vi "DualMotorControl_v2.vi"() -> ()   [LabVIEW 2019]
uses:
  <vilib>/myRIO/Common/Instrument Driver Framework/myRIO v1.0/Encoder/typedefs/Encoder Signal Mode.ctl
  <vilib>/myRIO/Instrument Drivers/Onboard IO/Encoder/typedefs/Encoder Reference.ctl
  <vilib>/myRIO/Common/Instrument Driver Framework/Utilities/typedefs/myRIO Generic Hardware Reference.ctl
  <vilib>/myRIO/Common/Instrument Driver Framework/Utilities/typedefs/Hardware Version Enum.ctl
  <vilib>/myRIO/Common/Instrument Driver Framework/Utilities/typedefs/myRIO v1.0 Reference.ctl
  <vilib>/myRIO/Common/Instrument Driver Framework/Utilities/typedefs/Generic FPGA Reference.ctl
  <vilib>/myRIO/Common/Instrument Driver Framework/myRIO v1.0/Encoder/typedefs/Encoder Channels Enum.ctl
  <vilib>/myRIO/Common/Instrument Driver Framework/myRIO v1.0/Encoder/typedefs/Encoder Configuration v1.0.ctl
  <vilib>/userDefined/High Color/nirio_resource_hc.ctl
  <vilib>/Platform/TimedLoop/XDataNode/timing_clust.ctl
  <vilib>/Platform/TimedLoop/XDataNode/nitl_modes.ctl
  <vilib>/Platform/TimedLoop/XDataNode/wakeup.ctl
  <vilib>/myRIO/Instrument Drivers/Onboard IO/PWM/typedefs/PWM Reference.ctl
  <vilib>/myRIO/Common/Instrument Driver Framework/myRIO v1.0/PWM/typedefs/PWM Channels Enum.ctl
  <vilib>/myRIO/Instrument Drivers/Onboard IO/PWM/typedefs/PWM Configuration.ctl
  <vilib>/myRIO/Instrument Drivers/Onboard IO/DIO/typedefs/DIO Reference.ctl
  <vilib>/myRIO/Common/Instrument Driver Framework/myRIO v1.0/DIO/typedefs/DIO Channels List.ctl
  <vilib>/myRIO/Common/Instrument Driver Framework/myRIO v1.0/DIO/typedefs/DIO Channels Enum.ctl
  <vilib>/myRIO/Common/Instrument Driver Framework/Utilities/vis/Is FPGA Ref Available.vi
  <vilib>/myRIO/Common/Instrument Driver Framework/myRIO v1.0/Encoder/vis/myRIO v1.1 Open Encoder.vi
  <vilib>/myRIO/Instrument Drivers/Onboard IO/Encoder/vis/Read.vi
  <vilib>/myRIO/Common/Instrument Driver Framework/myRIO v1.0/PWM/vis/myRIO v1.1 Open PWM.vi
  <vilib>/myRIO/Instrument Drivers/Onboard IO/PWM/vis/Set Duty Cycle and Frequency.vi
  <vilib>/myRIO/Common/Instrument Driver Framework/myRIO v1.0/DIO/vis/myRIO v1.1 Open DIO.vi
  <vilib>/myRIO/Instrument Drivers/Onboard IO/DIO/vis/Write.vi
  <vilib>/myRIO/Common/Instrument Driver Framework/Utilities/vis/Validate Channels.vi
  <vilib>/myRIO/Common/Instrument Driver Framework/myRIO v1.0/Encoder/vis/myRIO v1.0 Reserve Encoder.vi
  <vilib>/myRIO/Common/Instrument Driver Framework/myRIO v1.0/PWM/vis/myRIO v1.0 Reserve PWM.vi
  <vilib>/myRIO/Common/Instrument Driver Framework/myRIO v1.0/DIO/vis/myRIO v1.0 Reserve DIO.vi
  <vilib>/myRIO/Common/Instrument Driver Framework/myRIO v1.0/Encoder/vis/myRIO v1.0 Build MUX Configuration Encoder.vi
  <vilib>/myRIO/Common/Instrument Driver Framework/myRIO v1.0/Resource Manager/vis/myRIO v1.0 Reserve Channel List.vi
  <vilib>/myRIO/Common/Instrument Driver Framework/myRIO v1.0/PWM/vis/myRIO v1.0 Build MUX Configuration PWM.vi
  <vilib>/myRIO/Common/Instrument Driver Framework/myRIO v1.0/DIO/vis/myRIO v1.0 Build MUX Configuration DIO.vi
  <vilib>/myRIO/Common/Instrument Driver Framework/myRIO v1.0/Resource Manager/vis/myRIO v1.0 Create Configuration List.vi
  <vilib>/myRIO/Common/Instrument Driver Framework/myRIO v1.0/Resource Manager/vis/myRIO v1.0 Reserve Channel.vi
  <vilib>/myRIO/Common/Instrument Driver Framework/myRIO v1.0/Resource Manager/vis/myRIO v1.0 Unreserve Channel.vi
  <vilib>/myRIO/Common/Instrument Driver Framework/myRIO v1.0/Resource Manager/vis/myRIO v1.0 Build Mutex Name.vi
  <vilib>/Utility/VariantDataType/GetNumericInfo.vi
  <vilib>/Utility/error.llb/Error Cluster From Error Code.vi
  <vilib>/myRIO/Common/Instrument Driver Framework/myRIO v1.0/myRIO v1.1 Open.vi
  <vilib>/myRIO/Common/Instrument Driver Framework/Utilities/vis/IO Manager.vi
  <vilib>/myRIO/Common/Instrument Driver Framework/Utilities/vis/Configuration Manager.vi
  <vilib>/myRIO/Common/Instrument Driver Framework/myRIO v1.0/Resource Manager/vis/myRIO v1.0 Configure IO.vi
  <vilib>/myRIO/Common/Instrument Driver Framework/myRIO v1.0/myRIO v1.0 Close.vi
  <vilib>/myRIO/Common/Instrument Driver Framework/myRIO v1.0/Encoder/vis/myRIO v1.0 Configure Encoder.vi
  <vilib>/myRIO/Common/Instrument Driver Framework/myRIO v1.0/Encoder/vis/myRIO v1.0 Read Encoder.vi
  <vilib>/Instr/_visa.llb/VISA Configure Serial Port (Instr).vi
  <vilib>/myRIO/Common/Instrument Driver Framework/myRIO v1.0/PWM/vis/myRIO v1.0 Write PWM.vi
  <vilib>/myRIO/Common/Instrument Driver Framework/myRIO v1.0/DIO/vis/myRIO v1.0 Write DIO.vi
  <vilib>/Utility/file.llb/Write Delimited Spreadsheet (DBL).vi
  <vilib>/myRIO/Express VI/Onboard IO/Encoder/Encoder Express VI.xnode
  <vilib>/myRIO/Instrument Drivers/Onboard IO/Encoder/vis/myRIO Encoder Open.xnode
  <vilib>/myRIO/Common/Instrument Driver Framework/myRIO v1.0/Encoder/typedefs/Encoder Count Direction Enum.ctl
  <vilib>/Platform/TimedLoop/XDataNode/XDataNode.xnode
  <vilib>/myRIO/Express VI/Onboard IO/PWM/PWM Express VI.xnode
  <vilib>/myRIO/Instrument Drivers/Onboard IO/PWM/vis/myRIO PWM Open.xnode
  <vilib>/myRIO/Express VI/Onboard IO/DO/DO Express VI.xnode
  <vilib>/myRIO/Instrument Drivers/Onboard IO/DIO/vis/myRIO DIO Open.xnode
  <vilib>/myRIO/Instrument Drivers/Onboard IO/Encoder/Encoder.lvlib
  <vilib>/Platform/TimedLoop/XDataNode/XDNodeRunTimeDep.lvlib
  <vilib>/myRIO/Instrument Drivers/Onboard IO/PWM/PWM.lvlib
  <vilib>/myRIO/Instrument Drivers/Onboard IO/DIO/DIO.lvlib
panel:
  out "element":string
  in  "Encoder_Count":dbl=54991.0
  out "number":i32
  in  "text":string[](array[string])
  in  "start FIFO":bool=TRUE
  out "Write FIFO error":errorcluster
  out "# elements write":u32=219
  out "timed out?":bool
  out "rt fifo":refnum<k33>
  in  "Buffer factor":dbl=1.5
  out "# elements read":u32
  out "date/time string":string="1970011"
  out "Create FIFO error":errorcluster
  in  "Experiment Mode":string="20250310_servo_sinewave"
  in  "Times":string="0"
  in  "File Path Control":path=path "C:/Rhex_ABAD"
  out "error out":errorcluster
  in  "baud rate (9600)":u32=500000
  in  "VISA resource name":refnum<visa-resource-name>="ASRL2::INSTR"
  in  "stop":bool
  in  "const posotion":dbl=180.0
  out "write to visa":string
  out "read from visa":string
  out "sine position":dbl
  out "time":dbl
  out "iteration":i32
  in  "const(f)/sine(t)":bool
  in  "sinewave period":dbl=10.0
  in  "Gain":T1={"P Gain"=0.5, "I Gain"=0.0, "D Gain"=0.005}
  in  "Frequency":dbl=1000.0
  out "Duty cycle  2":dbl
  in  "Loop Period":i64=5
  # "Servo motor"
  # "Control botton"
  # "Plot"
  # "visa setting"
  # "servo setting"
  # "Timed loop status"
  # "DC motor"
  # "R-SLIP Parameters"
  # "v = 1; a = 15"
  # "v = 1.25; a = 15"
  # "v = 1.5; a = 15"
  # "0.184067181524967\n0.263820978418769\n256152.551336786\n-30272.30000274\n-9876.03760433421\n-1096.38594197941\n885.91817900106\n-44.6781799901984"
  # "0.215241998794118\n0.254514142390288\n4771.41078363533\n62185.8763006578\n-22508.5336527453\n390.805502041188\n686.695311017595\n-40.4128145310291"
  # "0.163616269216122\n0.27489641502463\n771965.39318528\n-201617.027694185\n8828.08396944145\n-2683.04589908678\n1085.57303422127\n-48.5860395324432"
  # "v = 1.75; a = 15"
  # "v = 2; a = 15"
  # "v = 2.25; a = 15"
  # "0.148651048423414\n0.288542414074344\n1776973.44893281\n-511591.467559457\n38775.9830765103\n-4576.94506688942\n1289.39828252671\n-52.3115561007577"
  # "0.136976185169818\n0.304016701267508\n3461279.85083822\n-993110.73746345\n80544.6579529191\n-6699.48295844177\n1494.82265451498\n-55.8934424469099"
  # "0.134381902205816\n0.369022171779704\n3272804.8365432\n-899365.569589567\n71225.2463409934\n-7039.10791102172\n1512.66147498591\n-59.3408899720725"
  # "FIFO status"
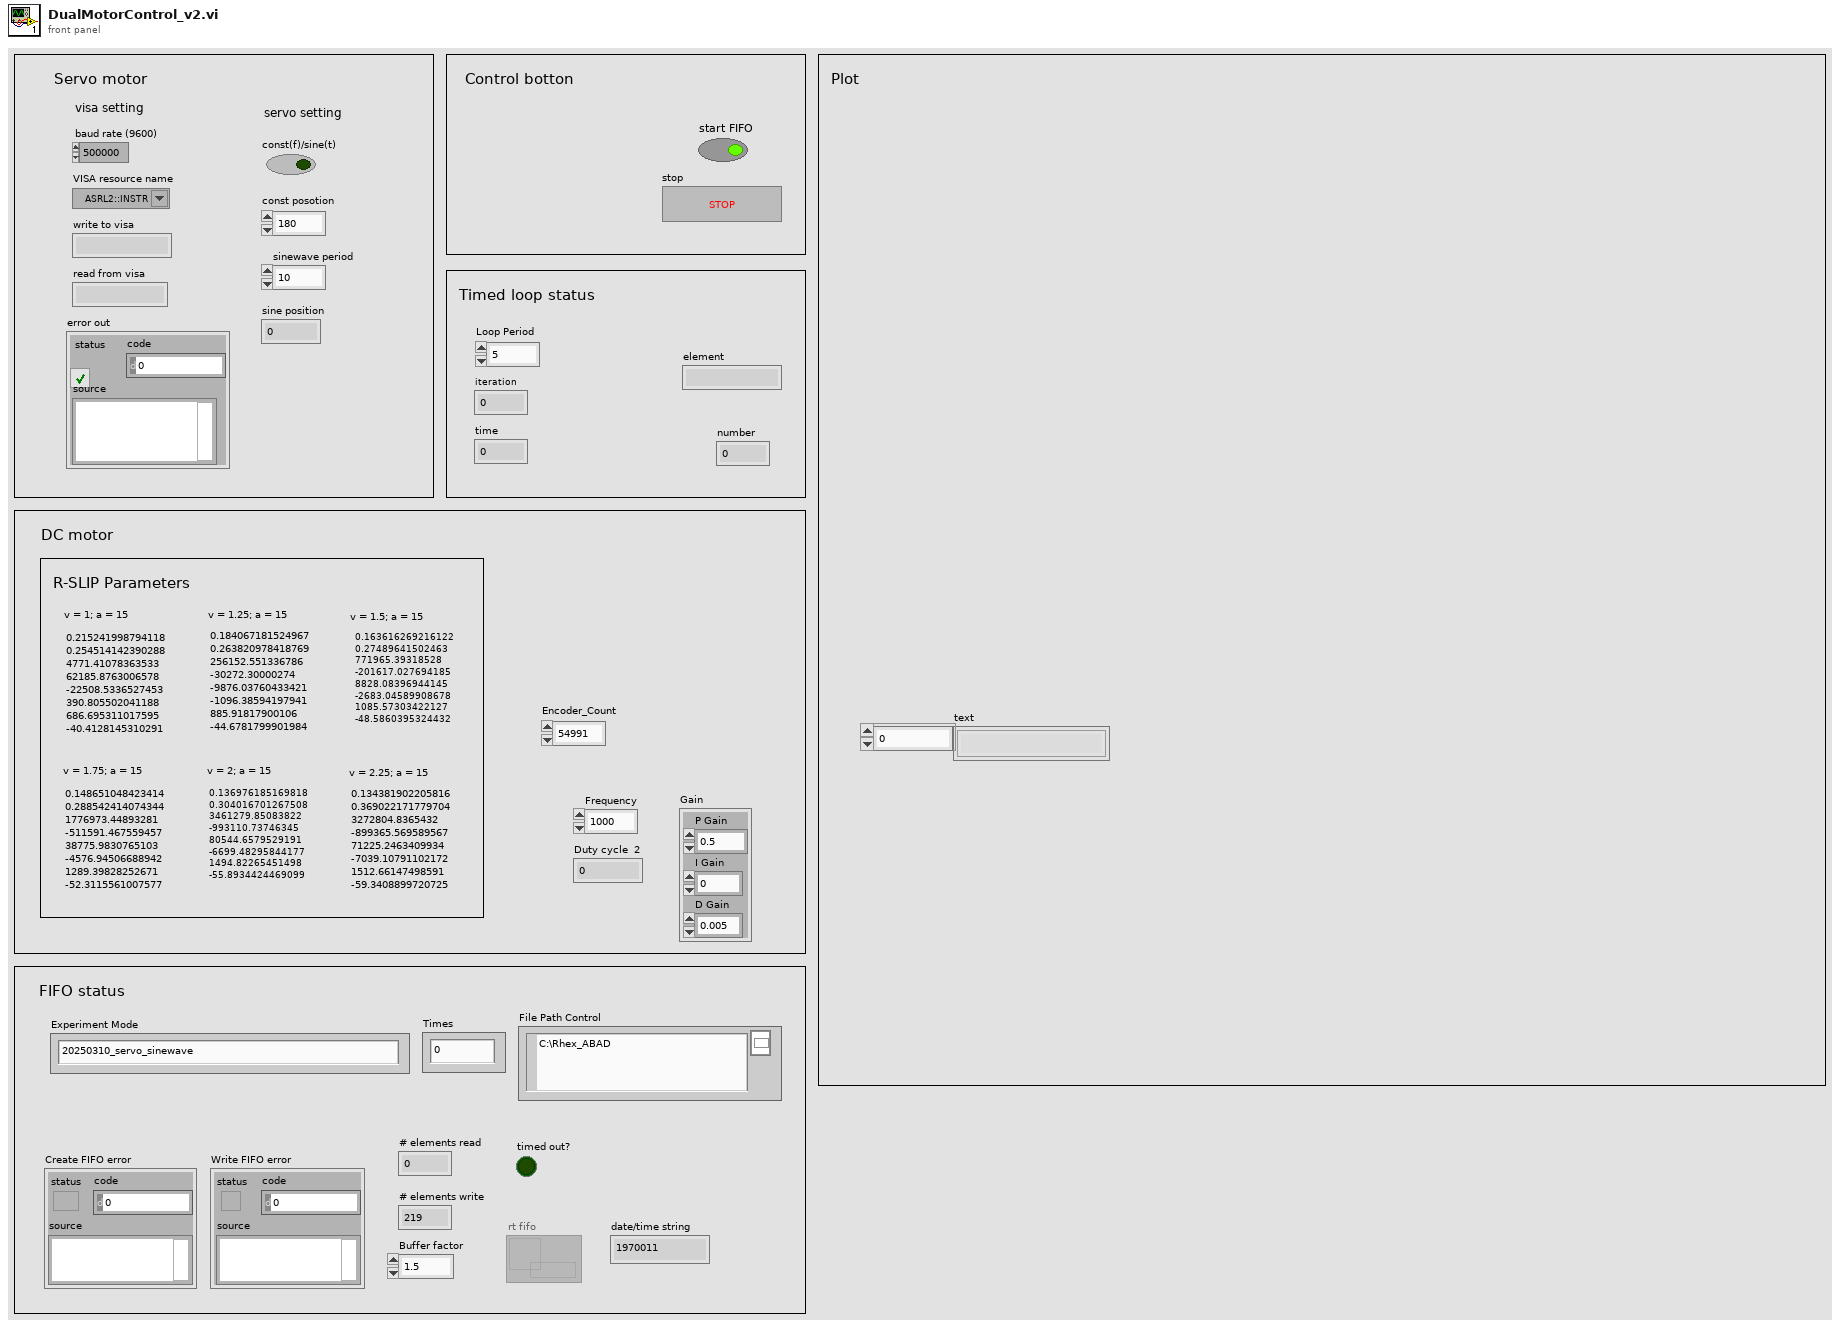
[diagram p1: front panel]
types:
  T1 = cluster{"P Gain":dbl, "I Gain":dbl, "D Gain":dbl}
  T2 = typedef "Encoder.lvlib/Encoder Reference.ctl" = cluster{"myRIO Reference":T3, "Encoder Channels Enum":T7}
  T3 = typedef "myRIO Generic Hardware Reference.ctl" = cluster{"myRIO Model":T4, "myRIO Hardware Reference":T5}
  T4 = typedef "Hardware Version Enum.ctl" = enum16{"Unknown", "myRIO-1900", "myRIO-1950", "roboRIO", "NI ELVIS RIO CM", "ELVIS III"}
  T5 = typedef "myRIO v1.0 Reference.ctl" = cluster{"Generic FPGA Reference":T6, "Allow multiple opens":bool}
  T6 = typedef "Generic FPGA Reference.ctl" = refnum<k20>
  T7 = typedef "Encoder Channels Enum.ctl" = enum16{"Not Connected", "C/ENC0", "C/ENC1", "A/ENC", "A/ENC0", "A/ENC1", "A/ENC2", "A/ENC3", "A/ENC4", "A/ENC5", "A/ENC6", "A/ENC7", "A/ENC8", "A/ENC9", "B/ENC", "B/ENC0", "B/ENC1", "B/ENC2", "B/ENC3", "B/ENC4", "B/ENC5", "B/ENC6", "B/ENC7", "B/ENC8", "B/ENC9", "DIO/ENC0", "DIO/ENC1", "DIO/ENC2", "DIO/ENC3", "DIO/ENC4"}
  T8 = typedef "Encoder Signal Mode.ctl" = enum16{"Quadrature phase signal", "Step and direction signal"}
  T9 = typedef "nirio_resource_hc.ctl" = tag
  T10 = typedef "DIO.lvlib/DIO Reference.ctl" = cluster{"myRIO Reference":T3, "DIO Channels List":T11}
  T11 = typedef "DIO Channels List.ctl" = T12[]
  T12 = typedef "DIO Channels Enum.ctl" = enum16{"Not Connected", "C/DIO0", "C/DIO1", "C/DIO2", "C/DIO3", "C/DIO4", "C/DIO5", "C/DIO6", "C/DIO7", "A/DIO0", "A/DIO1", "A/DIO2", "A/DIO3", "A/DIO4", "A/DIO5", "A/DIO6", "A/DIO7", "A/DIO8", "A/DIO9", "A/DIO10", "A/DIO11", "A/DIO12", "A/DIO13", "A/DIO14", "A/DIO15", "A/DIO16", "A/DIO17", "A/DIO18", "A/DIO19", "B/DIO0", "B/DIO1", "B/DIO2", "B/DIO3", "B/DIO4", "B/DIO5", "B/DIO6", "B/DIO7", "B/DIO8", "B/DIO9", "B/DIO10", "B/DIO11", "B/DIO12", "B/DIO13", "B/DIO14", "B/DIO15", "B/DIO16", "B/DIO17", "B/DIO18", "B/DIO19", "LED0", "LED1", "LED2", "LED3", "Button0", "DIO/DIO0", "DIO/DIO1", "DIO/DIO2", "DIO/DIO3", "DIO/DIO4", "DIO/DIO5", "DIO/DIO6", "DIO/DIO7", "DIO/DIO8", "DIO/DIO9", "SPI/CS0", "SPI/CS1", "SPI/CS2", "SPI/CS3", "LED RADIO (Green)", "LED RADIO (Red)", "LED COMM (Green)", "LED COMM (Red)", "LED MODE (Green)", "LED MODE (Red)"}
  T13 = typedef "PWM.lvlib/PWM Reference.ctl" = cluster{"myRIO Reference":T3, "PWM Channels Enum":T14, "PWM Configuration":T15}
  T14 = typedef "PWM Channels Enum.ctl" = enum16{"Not Connected", "C/PWM0", "C/PWM1", "A/PWM0", "A/PWM1", "A/PWM2", "A/PWM3", "A/PWM4", "A/PWM5", "A/PWM6", "A/PWM7", "A/PWM8", "A/PWM9", "A/PWM10", "A/PWM11", "A/PWM12", "A/PWM13", "A/PWM14", "A/PWM15", "A/PWM16", "A/PWM17", "A/PWM18", "A/PWM19", "B/PWM0", "B/PWM1", "B/PWM2", "B/PWM3", "B/PWM4", "B/PWM5", "B/PWM6", "B/PWM7", "B/PWM8", "B/PWM9", "B/PWM10", "B/PWM11", "B/PWM12", "B/PWM13", "B/PWM14", "B/PWM15", "B/PWM16", "B/PWM17", "B/PWM18", "B/PWM19", "PWM/PWM0", "PWM/PWM1", "PWM/PWM2", "PWM/PWM3", "PWM/PWM4", "PWM/PWM5", "PWM/PWM6", "PWM/PWM7", "PWM/PWM8", "PWM/PWM9"}
  T15 = typedef "PWM.lvlib/PWM Configuration.ctl" = cluster{"Frequency":dbl, "Duty Cycle":dbl}
  T16 = typedef "XDNodeRunTimeDep.lvlib/timing_clust.ctl" = cluster{"Expected End [f-1]":u64, "Actual End [f-1]":u64, "Finished Late? [f-1]":bool, "Expected End [i-1]":u64, "Actual End [i-1]":u64, "Finished Late? [i-1]":bool, "Expected Start [i]":u64, "Actual Start [i]":u64, "Expected Start [f]":u64, "Actual Start [f]":u64, "Source Name":string, "Structure Name":string, "Period":i64, "Deadline":i64, "Offset":i64, "Start":i64, "Priority":i32, "Timeout":i32, "Mode":T17, "Wakeup Reason":T18, "Error":errorcluster, "Source Type":string, "Secondary Source Type":string, "Global End Time":u64, "Global Start Time":u64, "Frame Duration":u64, "Iteration Duration":u64, "Assigned CPU":i32, "I/O Scan Engine Mode":u32}
  T17 = typedef "XDNodeRunTimeDep.lvlib/nitl_modes.ctl" = enum32{"No Change", "Process missed periods, maintain original phase", "Discard missed periods, maintain original phase", "Process missed periods, ignore original phase", "Discard missed periods, ignore original phase"}
  T18 = typedef "XDNodeRunTimeDep.lvlib/wakeup.ctl" = enum32{"Normal", "Aborted", "Asynchronous wakeup", "Timing source error", "Timed loop error", "Timeout"}
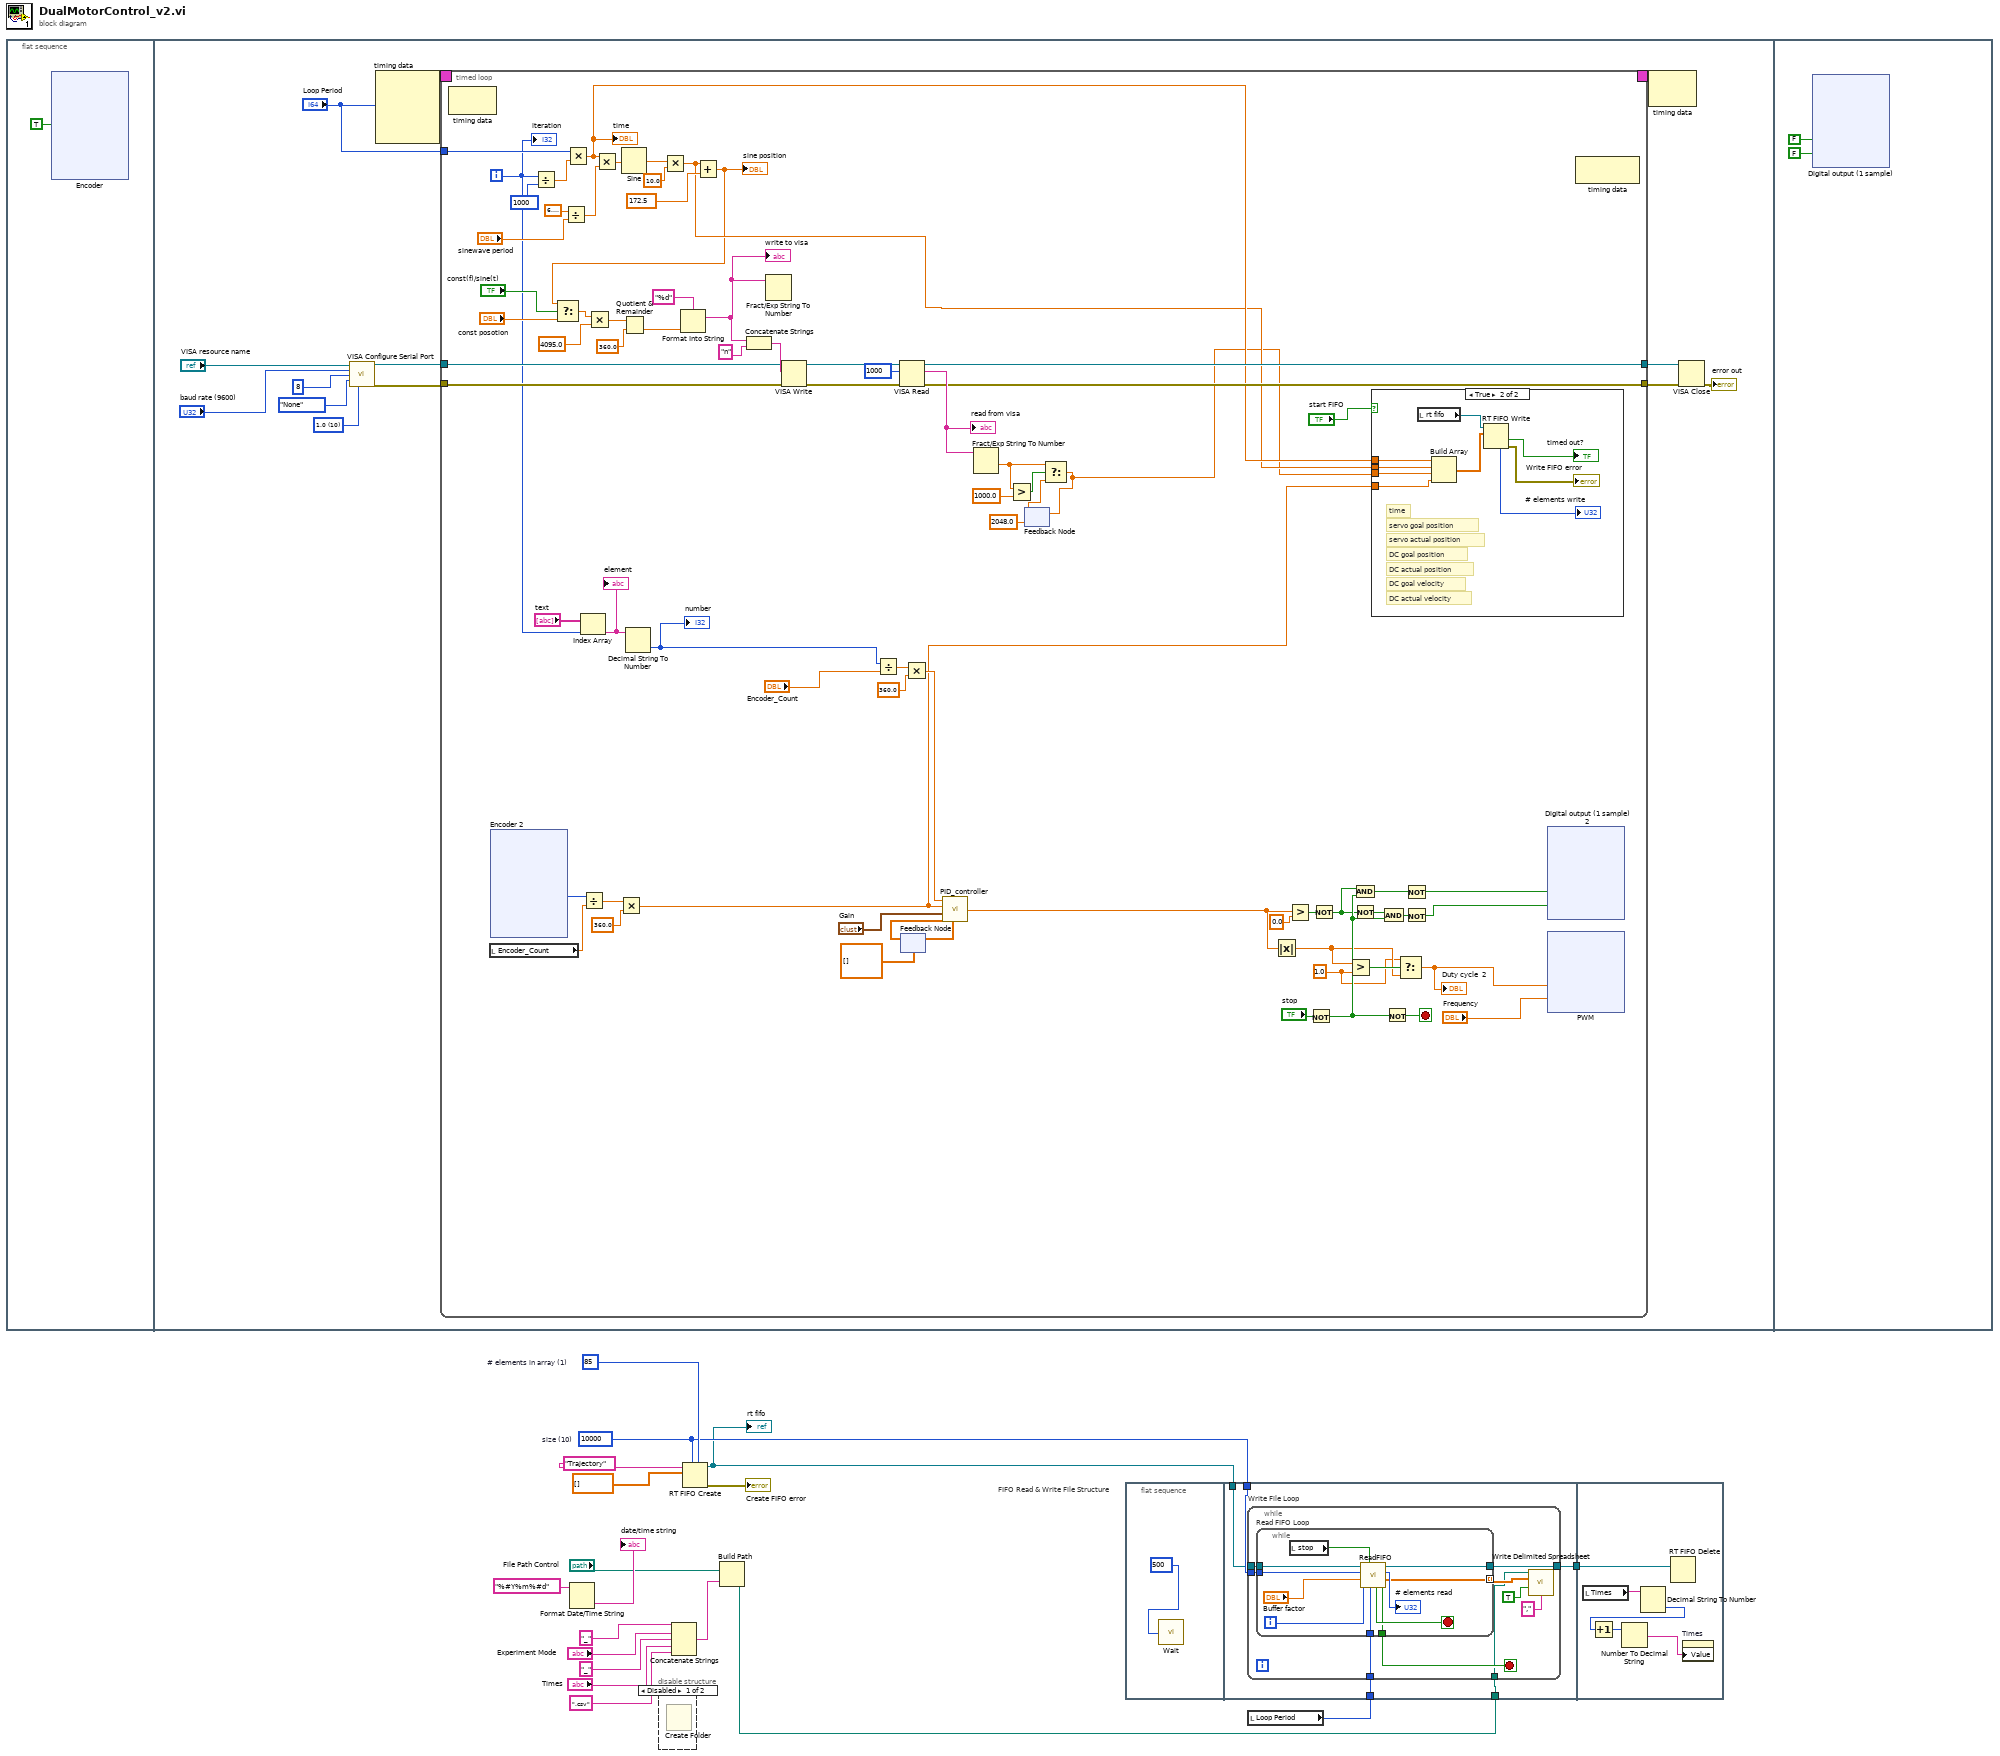
[diagram p0: block diagram]
diagram:
  w7 = u32 85  # # elements in array (1)
  w3 = u32 10000  # size (10)
  n1 = flat-sequence {
    frame #0 {
      n2 = xnode "Encoder"("Reset Counter"=TRUE) -> ()  [unwired: 1 in, 4 out]
    }
    frame #1 {
      w73 = u16 10 items=["1.0"=10, "1.5"=15, "2.0"=20] ("stop bits (10: 1 bit)")
      n3 = call-poly "VISA Configure Serial Port"("VISA resource name"="VISA resource name", "baud rate (9600)"="baud rate (9600)", "data bits (8)"=u16 8, "parity (0:none)"=enum16{"None", "Odd", "Even", "Mark", "Space"}."None", "stop bits (10: 1 bit)"=w73) -> ("VISA resource name out"=w72:refnum<visa-resource-name>, "error out"=w71:errorcluster)  [unwired: 9 in]
      n4 = node-c288("Loop Period") -> (w78:T16)  [unwired: 3 in]
      n5 = timed-loop {
        timing: w78 -> [_]
        timing-out: [_] -> w77
        tunnel: "Loop Period" -> [w130]
        tunnel: w71 -> [w131]
        tunnel: [w129] -> w70
        tunnel: w72 -> [w132]
        tunnel: [w128] -> w66
        i -> [w82]
        stop <- w98 stop-if-true
        w95 = 1.0 ("y")
        n6 = node-c288() -> ()  [unwired: 1 in, 1 out]
        n7 = local read "Encoder_Count"() -> (w119:dbl)
        n8 = xnode "Encoder 2"() -> ("Counter Value"=w118:i32)  [unwired: 2 in, 3 out]
        n9 = Divide(x=w82, y=i64 1000) -> (x/y=w139:dbl)
        n10 = Divide(x=6.283185307179586, y="sinewave period") -> (x/y=w122:dbl)
        n11 = Multiply(x=w130, y=w139) -> (x*y=w93:dbl)
        "time" <- w93
        n12 = Index Array(array="text", index=w82) -> (element=w81:string)
        "element" <- w81
        n13 = Divide(x=w118, y=w119) -> (x/y=w116:dbl)
        n14 = Multiply(x=w93, y=w122) -> (x*y=w142:dbl)
        n15 = Multiply(x=w116, y=360.0 ("x")) -> (x*y=w90:dbl)
        n16 = Sine(x=w142) -> (sin(x)=w136:dbl)
        n17 = Decimal String To Number(string=w81) -> (number=w79:i32)  [unwired: 2 in, 1 out]
        "number" <- w79
        n18 = Multiply(x=w136, y=10.0) -> (x*y=w92:dbl)
        n19 = Add(x=w92, y=172.5) -> (x+y=w89:dbl)
        "sine position" <- w89
        n20 = Select(t=w89, s="const(f)/sine(t)", f="const posotion") -> (s? t:f=w88:dbl)
        n21 = Multiply(x=w88, y=4095.0) -> (x*y=w149:dbl)
        n22 = Quotient & Remainder(x=w149, y=360.0) -> (floor(x/y)=w147:dbl)  [unwired: 1 out]
        n23 = Format Into String(format string="%d", w147) -> (resulting string=w143:string)  [unwired: 2 in, 1 out]
        "write to visa" <- w143
        n24 = Concatenate Strings(w143, "n" ("string")) -> (w151:string)
        n25 = Fract/Exp String To Number(string=w143) -> ()  [unwired: 3 in, 2 out]
        n26 = VISA Write(VISA resource name=w132, write buffer=w151, error in (no error)=w131) -> (VISA resource name out=w86:refnum<visa-resource-name>, error out=w85:errorcluster)  [unwired: 1 out]
        n27 = Divide(x=w79, y="Encoder_Count") -> (x/y=w121:dbl)
        n28 = VISA Read(VISA resource name=w86, byte count=u32 1000, error in (no error)=w85) -> (VISA resource name out=w128:refnum<visa-resource-name>, read buffer=w144:string, error out=w129:errorcluster)  [unwired: 1 out]
        "read from visa" <- w144
        n29 = feedback #1(dbl[] [] ("state(k)")) -> (w114:dbl[])
        n30 = Multiply(x=w121, y=360.0 ("x")) -> (x*y=w91:dbl)
        n31 = call "PID_controller.vi"("state(k-1)"=w114, "Gain"="Gain", "variable"=w90, "set point"=w91) -> ("PID gain"=w96:dbl, "state(k)"=w113:dbl[])  [unwired: 1 in]
        n32 = feedback-in #1(w113) -> ()
        n33 = Fract/Exp String To Number(string=w144) -> (number=w134:dbl)  [unwired: 3 in, 1 out]
        n34 = Greater?(x=w134, y=1000.0) -> (0:w133:bool)
        n35 = feedback #2(2048.0) -> (w126:dbl)
        n36 = Select(t=w134, s=w133, f=w126) -> (s? t:f=w87:dbl)
        n37 = feedback-in #2(w87) -> ()
        n38 = Absolute Value(x=w96) -> (abs(x)=w105:dbl)
        n39 = Greater?(x=w96, y=0.0) -> (0:w107:bool)
        n40 = Not(x="stop") -> (.not. x?=w109:bool)
        n41 = Not(x=w107) -> (.not. x?=w104:bool)
        n42 = Greater?(x=w105, y=w95) -> (0:w106:bool)
        n43 = And(x=w104, y=w109) -> (x .and. y?=w101:bool)
        n44 = Not(x=w104) -> (.not. x?=w110:bool)
        n45 = case shown="True" "start FIFO" {
          tunnel: w93 -> [_ w155]
          tunnel: w92 -> [_ w154]
          tunnel: w87 -> [_ w153]
          tunnel: w90 -> [_ w152]
          frame False {
          }
          frame True {
            # "DC actual velocity"
            # "DC goal velocity"
            # "DC actual position"
            # "DC goal position"
            # "time"
            # "servo actual position"
            # "servo goal position"
            n46 = local read "rt fifo"() -> (w157:refnum<k33>)
            n47 = Build Array(w155, w154, w153, w152) -> (w156:dbl[])
            n48 = RT FIFO Write(0:w157, 1:w156) -> (7:→"# elements write":u32, 10:→"timed out?":bool, 11:→"Write FIFO error":errorcluster)  [unwired: 3 in, 1 out]
          }
        }
        n49 = And(x=w110, y=w109) -> (x .and. y?=w103:bool)
        n50 = Not(x=w109) -> (.not. x?=w98:bool)
        n51 = Select(t=w95, s=w106, f=w105) -> (s? t:f=w99:dbl)
        "Duty cycle  2" <- w99
        n52 = Not(x=w101) -> (.not. x?=w100:bool)
        n53 = Not(x=w103) -> (.not. x?=w102:bool)
        n54 = xnode "Digital output (1 sample) 2"("A/DIO0 (Pin 11)"=w100, "A/DIO1 (Pin 13)"=w102) -> ()  [unwired: 1 in, 1 out]
        n55 = xnode "PWM"("Duty Cycle"=w99, "Frequency [Hz]"="Frequency") -> ()  [unwired: 1 in, 1 out]
        n56 = node-c288() -> ()  [unwired: 1 in, 1 out]
        "iteration" <- w82
      }
      n57 = node-c288(w77) -> ()  [unwired: 1 out]
      n58 = VISA Close(VISA resource name=w66, error in (no error)=w70) -> (error out=→"error out":errorcluster)
    }
    frame #2 {
      n59 = xnode "Digital output (1 sample)"("A/DIO0 (Pin 11)"=FALSE, "A/DIO1 (Pin 13)"=FALSE) -> ()  [unwired: 1 in, 1 out]
    }
  }
  n60 = Format Date/Time String(time format string (%c)="%#Y%m%#d" ("String 2")) -> (date/time string=→"date/time string":string)  [unwired: 2 in]
  n61 = disable-structure shown="Disabled" {
    frame Disabled {
      n62 = Create Folder() -> ()  [unwired: 3 in, 3 out]
    }
    frame Enabled {
    }
  }
  n63 = Concatenate Strings("_" ("String 2"), "Experiment Mode", "_" ("String 2"), "Times", ".csv" ("string")) -> (w11:string)
  n64 = RT FIFO Create(0:"Trajectory" ("name (unnamed)"), 1:dbl[] [], 4:w3, 6:w7) -> (8:w2:refnum<k33>, 11:→"Create FIFO error":errorcluster)  [unwired: 4 in, 1 out]
  "rt fifo" <- w2
  n65 = Build Path(base path="File Path Control", name or relative path=w11) -> (appended path=w9:path)
  n66 = flat-sequence "FIFO Read & Write File Structure" {
    tunnel: w3 -> [w326]
    tunnel: w1 -> [w325]
    tunnel: w9 -> [w324]
    tunnel: w2 -> [w323]
    tunnel: [w327] -> w18
    tunnel: w18 -> [w348]
    frame #0 {
      n67 = call "Wait"("Count(mSec)"=u32 500 ("Count(uSec)")) -> ()  [unwired: 1 out]
    }
    frame #1 {
      n68 = while "Write File Loop" {
        tunnel: w323 -> [w336]
        tunnel: [w335] -> w327
        tunnel: w326 -> [w334]
        tunnel: w325 -> [w333]
        tunnel: w324 -> [w328]
        stop <- w332 stop-if-true
        n69 = while "Read FIFO Loop" {
          tunnel: w336 -> [w346]
          tunnel: [w340] -> w335
          tunnel: w334 -> [w345]
          tunnel: w333 -> [w343]
          tunnel: [w341] -> w332
          tunnel: [w338] -> w329 mode=indexing
          i -> [w337]
          stop <- w342 stop-if-true
          n70 = local read "stop"() -> (w347:bool)
          n71 = call "ReadFIFO.vi"("dt of Timeloop(ms)"=w343, "Stop"=w347, "Count"=w337, "Buffer factor"="Buffer factor", "FIFO size"=w345, "RT FIFO"=w346) -> ("Stop write file"=w341:bool, "element out"=w338:dbl[], "# elements"=→"# elements read":u32, "RT FIFO (to delete)"=w340:refnum<k33>, "Stop read file"=w342:bool)  [unwired: 1 in]
        }
        n72 = call-poly <vilib>:"Write Delimited Spreadsheet.vi"("file path (dialog if empty)"=w328, "2D data"=w329, "append to file? (new file:F)"=TRUE, "delimiter (\\t)"="," ("delimiter (\\t)")) -> ()  [unwired: 10 in, 2 out]
      }
    }
    frame #2 {
      n73 = local read "Times"() -> (w350:string)
      n74 = Decimal String To Number(string=w350) -> (number=w352:i32)  [unwired: 2 in, 1 out]
      n75 = Increment(x=w352) -> (x+1=w351:i32)
      n76 = Number To Decimal String(number=w351) -> (decimal integer string=w349:string)  [unwired: 1 in]
      n77 = RT FIFO Delete(0:w348) -> ()  [unwired: 2 in, 1 out]
      n78 = property on="Times" class="Str"("Value"=w349) -> ()  [unwired: 2 in, 2 out]
    }
  }
  n79 = local read "Loop Period"() -> (w1:i64)
